vi "Start or stop continuous status updates.vi"(8 "error in (no error)":errorcluster, 10 "Continuous status updates":bool, 11 "PS Control Actor in":refnum<class "PS Control Actor.lvclass">) -> (0 "error out":errorcluster, 3 "PS Control Actor out":refnum<class "PS Control Actor.lvclass">)   [LabVIEW 2019, in "PS Control Actor.lvlib" / "PS Control Actor.lvclass"]
uses:
  PS Control Actor.lvclass
  Applications/National Instruments/LabVIEW 2019 64-bit/vi.lib/ActorFramework/Actor/Actor.lvclass
  PS Control Actor.lvclass/PS Control Actor.ctl
  <vilib>/ActorFramework/Actor/Actor.lvclass/Actor.ctl
  <vilib>/ActorFramework/Message Enqueuer/Message Enqueuer.lvclass/Message Enqueuer.ctl
  <vilib>/ActorFramework/Message Enqueuer/Init from Existing Queue.vi
  <vilib>/ActorFramework/Message Enqueuer/Enqueue.vi
  PS Control Actor Messages/Get PS Status Msg/Get PS Status Msg.lvclass
  Applications/National Instruments/LabVIEW 2019 64-bit/vi.lib/ActorFramework/Message/Message.lvclass
  <vilib>/ActorFramework/Message Priority Queue/Priority Enqueue.vi
  <vilib>/ActorFramework/Message Enqueuer/Message Enqueuer.lvclass
  <vilib>/ActorFramework/Actor/Actor.lvclass
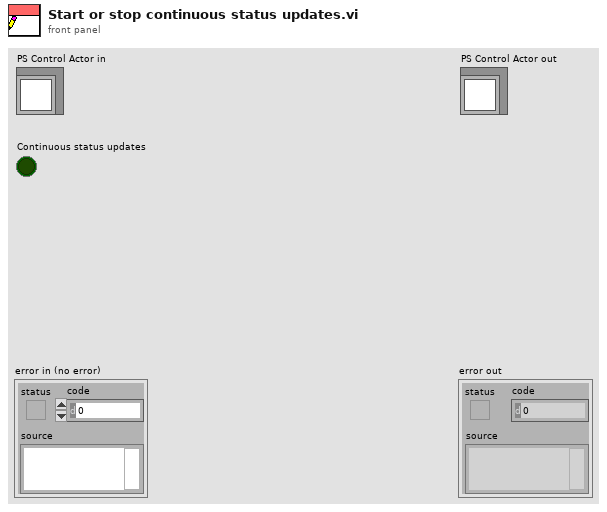
[diagram p1: front panel]
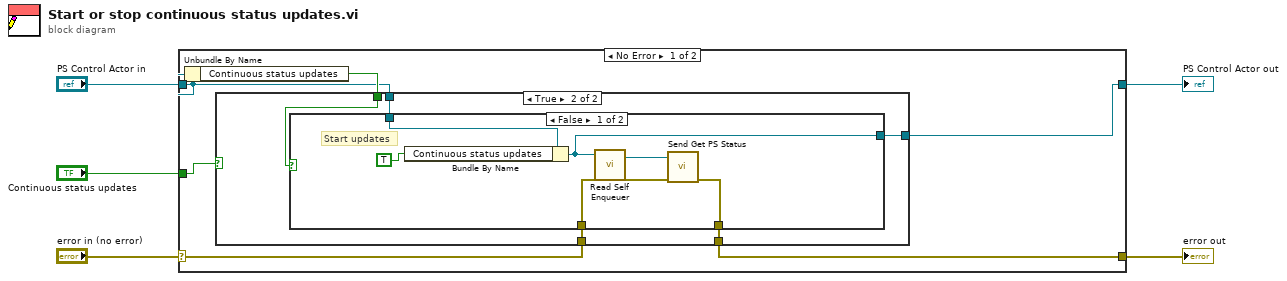
[diagram p0: block diagram]
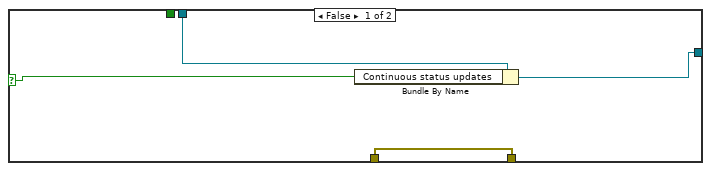
[diagram p2: hidden frame]
diagram:
  n1 = case shown="No Error" "error in (no error)" {
    selector: "error in (no error)" -> [w9 w29]
    tunnel: [w8 w29] -> w4
    tunnel: [w6 w30] -> w2
    tunnel: "PS Control Actor in" -> [w7 w30]
    tunnel: "Continuous status updates" -> [w11 _]
    frame No Error {
      n2 = Unbundle By Name(w7) -> ("Continuous status updates"=w10:bool)
      n3 = case shown="True" w11 {
        selector: w11 -> [w12 _]
        tunnel: w10 -> [_ w20]
        tunnel: w7 -> [w13 w19]
        tunnel: w9 -> [w15 w18]
        tunnel: [w15 w17] -> w8
        tunnel: [w14 w16] -> w6
        frame False {
          n4 = Bundle By Name(cluster=w13, "Continuous status updates"=w12) -> (w14:refnum<class "PS Control Actor.lvclass">)
        }
        frame True {
          n5 = case shown="False" w20 {
            tunnel: w19 -> [w23 w27]
            tunnel: w18 -> [w25 w28]
            tunnel: [w24 w28] -> w17
            tunnel: [w22 w27] -> w16
            frame False {
              # "Start updates"
              n6 = Bundle By Name(cluster=w23, "Continuous status updates"=TRUE) -> (w22:refnum<class "PS Control Actor.lvclass">)
              n7 = call <vilib>:"Read Self Enqueuer.vi"("Actor"=w22) -> ("Self Enqueuer"=w26:refnum<class "Message Enqueuer.lvclass">)  [unwired: 10 in]
              n8 = call "Send Get PS Status.vi"("error in (no error)"=w25, "Message Enqueuer"=w26) -> ("error out"=w24:errorcluster)  [unwired: 8 in, 1 out]
            }
            frame True {
              # "Already running. No change."
            }
          }
        }
      }
    }
    frame Error {
    }
  }
  "error out" <- w4
  "PS Control Actor out" <- w2
